vi "polarity_example.vi"() -> ()   [LabVIEW 2009]
panel:
  in  "Enum":enum32{"positive", "negative"}(ring)
  out "error out":errorcluster
  in  "error in (no error)":errorcluster
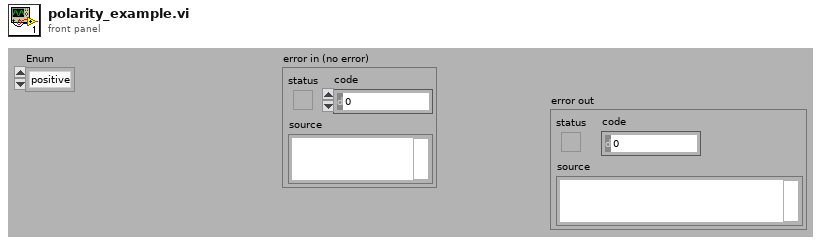
[diagram p1: front panel]
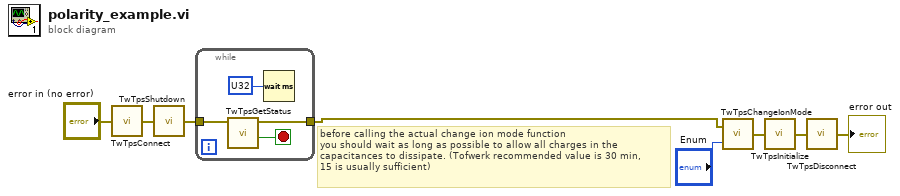
[diagram p0: block diagram]
diagram:
  # "before calling the actual change ion mode function\nyou should wait as long as possible to allow all charges in the \ncapacitances to dissipate. (Tofwerk recommended value is 30 min,\n15 is usually sufficient)"
  n1 = call "TwTpsConnect.vi"("error in (no error)"="error in (no error)") -> ("error out"=w6:errorcluster)
  n2 = call "TwTpsShutdown.vi"("error in (no error)"=w6) -> ("error out"=w5:errorcluster)
  n3 = while {
    tunnel: w5 -> [w11]
    tunnel: [w9] -> w4
    stop <- w10 stop-if-true
    n4 = call "TwTpsGetStatus.vi"("error in (no error)"=w11) -> ("canChangeIonMode?"=w10:bool, "error out"=w9:errorcluster)  [unwired: 5 out]
    n5 = Wait (ms)(milliseconds to wait=u32 ?) -> ()  [unwired: 1 out]
  }
  n6 = call "TwTpsChangeIonMode.vi"("Enum"="Enum", "error in (no error)"=w4) -> ("error out"=w2:errorcluster)
  n7 = call "TwTpsInitialize.vi"("error in (no error)"=w2) -> ("error out"=w1:errorcluster)
  n8 = call "TwTpsDisconnect.vi"("error in (no error)"=w1) -> ("error out"=→"error out":errorcluster)
